vi "Main Tclk.vi"() -> ()   [LabVIEW 2018] (continued)
                      frame 2 {
                        n2570 = local read "Specimen I array"() -> (w7608:sgl[])
                        n2571 = local read "Beam Dump 1 array"() -> (w7591:sgl[])
                        n2572 = local read "Milling I array"() -> (w7579:sgl[])
                        n2573 = call "Auto limits.vi"("Minimum half range"=0.5, "# of interquartile range or stdev"=6.0 ("# of sigma"), "Length"=100, "Input array"=w7608) -> ("Low limit"=w7606:dbl, "High limit"=w7607:dbl)  [unwired: 5 in, 1 out]
                        n2574 = call "Auto limits.vi"("Minimum half range"=0.5, "# of interquartile range or stdev"=6.0 ("# of sigma"), "Length"=100, "Input array"=w7591) -> ("Low limit"=w7593:dbl, "High limit"=w7592:dbl)  [unwired: 5 in, 1 out]
                        n2575 = call "Auto limits.vi"("Minimum half range"=0.5, "# of interquartile range or stdev"=6.0 ("# of sigma"), "Length"=100, "Input array"=w7579) -> ("Low limit"=w7581:dbl, "High limit"=w7580:dbl)  [unwired: 5 in, 1 out]
                        n2576 = To Single Precision Float(number=w7607) -> (single precision float=w7601:sgl)
                        n2577 = To Single Precision Float(number=w7606) -> (single precision float=w7600:sgl)
                        n2578 = To Single Precision Float(number=w7592) -> (single precision float=w7598:sgl)
                        n2579 = To Single Precision Float(number=w7593) -> (single precision float=w7599:sgl)
                        n2580 = To Single Precision Float(number=w7580) -> (single precision float=w7586:sgl)
                        n2581 = To Single Precision Float(number=w7581) -> (single precision float=w7587:sgl)
                        n2582 = local read "Specimen I high limit array"() -> (w7603:sgl[])
                        n2583 = local read "Specimen I low limit array"() -> (w7604:sgl[])
                        n2584 = local read "BD1 high limit array"() -> (w7596:sgl[])
                        n2585 = local read "Milling I high limit array"() -> (w7584:sgl[])
                        n2586 = local read "BD1 low limit array"() -> (w7595:sgl[])
                        n2587 = local read "Milling I low limit array"() -> (w7583:sgl[])
                        n2588 = Build Array (concatenate)(w7603, w7601) -> (w7602:sgl[])
                        n2589 = Build Array (concatenate)(w7604, w7600) -> (w7605:sgl[])
                        n2590 = Build Array (concatenate)(w7596, w7598) -> (w7597:sgl[])
                        n2591 = Build Array (concatenate)(w7595, w7599) -> (w7594:sgl[])
                        n2592 = Build Array (concatenate)(w7584, w7586) -> (w7585:sgl[])
                        n2593 = Build Array (concatenate)(w7583, w7587) -> (w7582:sgl[])
                        n2594 = local write "Specimen I high limit array"(w7602) -> ()
                        n2595 = local write "Specimen I low limit array"(w7605) -> ()
                        n2596 = local write "BD1 high limit array"(w7597) -> ()
                        n2597 = local write "Milling I high limit array"(w7585) -> ()
                        n2598 = local write "BD1 low limit array"(w7594) -> ()
                        n2599 = local write "Milling I low limit array"(w7582) -> ()
                      }
                      frame 3 {
                        n2600 = local read "Specimen I array"() -> (w7644:sgl[])
                        n2601 = local read "Beam Dump 1 array"() -> (w7627:sgl[])
                        n2602 = local read "Beam Dump 2 array"() -> (w7620:sgl[])
                        n2603 = call "Auto limits.vi"("Minimum half range"=0.5, "# of interquartile range or stdev"=6.0 ("# of sigma"), "Length"=100, "Input array"=w7644) -> ("Low limit"=w7642:dbl, "High limit"=w7643:dbl)  [unwired: 5 in, 1 out]
                        n2604 = call "Auto limits.vi"("Minimum half range"=0.5, "# of interquartile range or stdev"=6.0 ("# of sigma"), "Length"=100, "Input array"=w7627) -> ("Low limit"=w7629:dbl, "High limit"=w7628:dbl)  [unwired: 5 in, 1 out]
                        n2605 = call "Auto limits.vi"("Minimum half range"=0.5, "# of interquartile range or stdev"=6.0 ("# of sigma"), "Length"=100, "Input array"=w7620) -> ("Low limit"=w7618:dbl, "High limit"=w7619:dbl)  [unwired: 5 in, 1 out]
                        n2606 = To Single Precision Float(number=w7643) -> (single precision float=w7637:sgl)
                        n2607 = To Single Precision Float(number=w7642) -> (single precision float=w7636:sgl)
                        n2608 = To Single Precision Float(number=w7628) -> (single precision float=w7634:sgl)
                        n2609 = To Single Precision Float(number=w7629) -> (single precision float=w7635:sgl)
                        n2610 = To Single Precision Float(number=w7619) -> (single precision float=w7613:sgl)
                        n2611 = To Single Precision Float(number=w7618) -> (single precision float=w7612:sgl)
                        n2612 = local read "Specimen I high limit array"() -> (w7639:sgl[])
                        n2613 = local read "Specimen I low limit array"() -> (w7640:sgl[])
                        n2614 = local read "BD1 high limit array"() -> (w7632:sgl[])
                        n2615 = local read "BD2 high limit array"() -> (w7615:sgl[])
                        n2616 = local read "BD1 low limit array"() -> (w7631:sgl[])
                        n2617 = local read "BD2 low limit array"() -> (w7616:sgl[])
                        n2618 = Build Array (concatenate)(w7639, w7637) -> (w7638:sgl[])
                        n2619 = Build Array (concatenate)(w7640, w7636) -> (w7641:sgl[])
                        n2620 = Build Array (concatenate)(w7632, w7634) -> (w7633:sgl[])
                        n2621 = Build Array (concatenate)(w7631, w7635) -> (w7630:sgl[])
                        n2622 = Build Array (concatenate)(w7615, w7613) -> (w7614:sgl[])
                        n2623 = Build Array (concatenate)(w7616, w7612) -> (w7617:sgl[])
                        n2624 = local write "Specimen I high limit array"(w7638) -> ()
                        n2625 = local write "Specimen I low limit array"(w7641) -> ()
                        n2626 = local write "BD1 high limit array"(w7633) -> ()
                        n2627 = local write "BD2 high limit array"(w7614) -> ()
                        n2628 = local write "BD1 low limit array"(w7630) -> ()
                        n2629 = local write "BD2 low limit array"(w7617) -> ()
                      }
                      frame 100, Default {
                        n2630 = local read "Specimen I array"() -> (w7692:sgl[])
                        n2631 = local read "Beam Dump 1 array"() -> (w7675:sgl[])
                        n2632 = local read "Beam Dump 2 array"() -> (w7668:sgl[])
                        n2633 = local read "Milling I array"() -> (w7651:sgl[])
                        n2634 = call "Auto limits.vi"("Minimum half range"=0.5, "# of interquartile range or stdev"=6.0 ("# of sigma"), "Length"=100, "Input array"=w7692) -> ("Low limit"=w7690:dbl, "High limit"=w7691:dbl)  [unwired: 5 in, 1 out]
                        n2635 = call "Auto limits.vi"("Minimum half range"=0.5, "# of interquartile range or stdev"=6.0 ("# of sigma"), "Length"=100, "Input array"=w7675) -> ("Low limit"=w7677:dbl, "High limit"=w7676:dbl)  [unwired: 5 in, 1 out]
                        n2636 = call "Auto limits.vi"("Minimum half range"=0.5, "# of interquartile range or stdev"=6.0 ("# of sigma"), "Length"=100, "Input array"=w7668) -> ("Low limit"=w7666:dbl, "High limit"=w7667:dbl)  [unwired: 5 in, 1 out]
                        n2637 = call "Auto limits.vi"("Minimum half range"=0.5, "# of interquartile range or stdev"=6.0 ("# of sigma"), "Length"=100, "Input array"=w7651) -> ("Low limit"=w7653:dbl, "High limit"=w7652:dbl)  [unwired: 5 in, 1 out]
                        n2638 = To Single Precision Float(number=w7691) -> (single precision float=w7685:sgl)
                        n2639 = To Single Precision Float(number=w7690) -> (single precision float=w7684:sgl)
                        n2640 = To Single Precision Float(number=w7676) -> (single precision float=w7682:sgl)
                        n2641 = To Single Precision Float(number=w7677) -> (single precision float=w7683:sgl)
                        n2642 = To Single Precision Float(number=w7667) -> (single precision float=w7661:sgl)
                        n2643 = To Single Precision Float(number=w7666) -> (single precision float=w7660:sgl)
                        n2644 = To Single Precision Float(number=w7652) -> (single precision float=w7658:sgl)
                        n2645 = To Single Precision Float(number=w7653) -> (single precision float=w7659:sgl)
                        n2646 = local read "Specimen I high limit array"() -> (w7687:sgl[])
                        n2647 = local read "Specimen I low limit array"() -> (w7688:sgl[])
                        n2648 = local read "BD1 high limit array"() -> (w7680:sgl[])
                        n2649 = local read "BD2 high limit array"() -> (w7663:sgl[])
                        n2650 = local read "Milling I high limit array"() -> (w7656:sgl[])
                        n2651 = local read "BD1 low limit array"() -> (w7679:sgl[])
                        n2652 = local read "BD2 low limit array"() -> (w7664:sgl[])
                        n2653 = local read "Milling I low limit array"() -> (w7655:sgl[])
                        n2654 = Build Array (concatenate)(w7687, w7685) -> (w7686:sgl[])
                        n2655 = Build Array (concatenate)(w7688, w7684) -> (w7689:sgl[])
                        n2656 = Build Array (concatenate)(w7680, w7682) -> (w7681:sgl[])
                        n2657 = Build Array (concatenate)(w7679, w7683) -> (w7678:sgl[])
                        n2658 = Build Array (concatenate)(w7663, w7661) -> (w7662:sgl[])
                        n2659 = Build Array (concatenate)(w7664, w7660) -> (w7665:sgl[])
                        n2660 = Build Array (concatenate)(w7656, w7658) -> (w7657:sgl[])
                        n2661 = Build Array (concatenate)(w7655, w7659) -> (w7654:sgl[])
                        n2662 = local write "Specimen I high limit array"(w7686) -> ()
                        n2663 = local write "Specimen I low limit array"(w7689) -> ()
                        n2664 = local write "BD1 high limit array"(w7681) -> ()
                        n2665 = local write "BD2 high limit array"(w7662) -> ()
                        n2666 = local write "Milling I high limit array"(w7657) -> ()
                        n2667 = local write "BD1 low limit array"(w7678) -> ()
                        n2668 = local write "BD2 low limit array"(w7665) -> ()
                        n2669 = local write "Milling I low limit array"(w7654) -> ()
                      }
                    }
                  }
                }
                n2670 = local read "Delta X array for stop limit"() -> (w7442:sgl[])
                n2671 = local read "Delta Y array for stop limit"() -> (w7439:sgl[])
                n2672 = local read "X shift (nm/image)"() -> (w7428:sgl)
                n2673 = local read "Y shift (nm/image)"() -> (w7425:sgl)
                n2674 = Absolute Value(x=w7442) -> (abs(x)=w7435:sgl[])
                n2675 = Absolute Value(x=w7439) -> (abs(x)=w7434:sgl[])
                n2676 = local read "Delta X stop limit array"() -> (w7443:sgl[])
                n2677 = local read "Delta Y stop limit array"() -> (w7437:sgl[])
                n2678 = call "Auto limits.vi"("Method"="mean & stdev", "Minimum half range"=10.0 ("# of sigma"), "# of interquartile range or stdev"=6.0 ("# of sigma"), "Length"=10, "Input array"=w7435) -> ("High limit"=w7422:dbl)  [unwired: 4 in, 2 out]
                n2679 = call "Auto limits.vi"("Method"="mean & stdev", "Minimum half range"=10.0 ("# of sigma"), "# of interquartile range or stdev"=6.0 ("# of sigma"), "Length"=100, "Input array"=w7434) -> ("High limit"=w7438:dbl)  [unwired: 4 in, 2 out]
                n2680 = To Single Precision Float(number=w7422) -> (single precision float=w7445:sgl)
                n2681 = To Single Precision Float(number=w7438) -> (single precision float=w7424:sgl)
                n2682 = Absolute Value(x=w7428) -> (abs(x)=w7420:sgl)
                n2683 = Absolute Value(x=w7425) -> (abs(x)=w7421:sgl)
                n2684 = Add(x=w7445, y=w7420) -> (x+y=w7429:sgl)
                n2685 = Add(x=w7424, y=w7421) -> (x+y=w7426:sgl)
                n2686 = Build Array (concatenate)(w7443, w7429) -> (w7444:sgl[])
                n2687 = Build Array (concatenate)(w7437, w7426) -> (w7436:sgl[])
                n2688 = local write "Delta X stop limit array"(w7444) -> ()
                n2689 = local write "Delta Y stop limit array"(w7436) -> ()
              }
              frame #27 {
                n2690 = local read "Pause for reheat"() -> (w7722:bool)
                n2691 = local read "Auto re-engage"() -> (w7721:bool)
                n2692 = case shown="True" w7722 {
                  tunnel: w7721 -> [_ w7723]
                  frame False {
                  }
                  frame True {
                    n2693 = case shown="False" w7723 {
                      frame False {
                        n2694 = stacked-sequence {
                          frame #0 {
                            n2695 = local read "3D FIB-SEM Files"() -> (w7729:path)
                            n2696 = local read "Re-engage Files"() -> (w7732:path)
                            n2697 = Build Path(base path=w7729, name or relative path="LG low res.png " ("command line")) -> (appended path=w7728:path)
                            n2698 = Build Path(base path=w7732, name or relative path="pre.png " ("command line")) -> (appended path=w7727:path)
                            n2699 = Copy(9:TRUE ("run minimized? (F)"), 10:w7727, 11:w7728) -> ()  [unwired: 2 in, 3 out]
                          }
                          frame #1 {
                            n2700 = shared-variable ".\\Zeiss Library.lvlib\\Timestamp"() -> (→"Pre-reheat time":timestamp)  [unwired: 1 in, 1 out]
                            n2701 = local read "Last good FI"() -> (→"Pre-reheat FI":sgl)
                          }
                          frame #2 {
                            n2702 = local read "SEM Scan Parameters"() -> (w7735:T26)
                            n2703 = Unbundle By Name(w7735) -> ("X center (um)"=→"Pre-reheat X center (um)":sgl, "Y center (um)"=→"Pre-reheat Y center (um)":sgl, "Y stig"=w7738:sgl[][])
                            n2704 = local write "Pre-reheat Y stig"(w7738) -> ()
                          }
                        }
                      }
                      frame True {
                      }
                    }
                    n2705 = local write "Mill Manual Pause"(TRUE ("Mill Stop")) -> ()
                    n2706 = property on="Mill Manual Pause" class="Bool (strict)"("DisabledEnum"=T44."Disabled and Grayed Out" ("Disabled")) -> ()  [unwired: 2 in, 2 out]
                  }
                }
              }
              frame #28 {
                n2707 = local read "FIB"() -> (w7747:bool)
                n2708 = local read "Alert Settings"() -> (w7745:T36)
                n2709 = local read "Log time array"() -> (w7740:u32[])
                n2710 = case shown="True" w7747 {
                  frame False {
                  }
                  frame True {
                    n2711 = local read "Temp (F)"() -> (w7798:sgl)
                    n2712 = local read "Faraday Cup (nA)"() -> (w7799:sgl)
                    n2713 = local read "Specimen I (nA)"() -> (w7800:sgl)
                    n2714 = local read "Beam Dump 1 (nA)"() -> (w7801:sgl)
                    n2715 = local read "Beam Dump 2 (nA)"() -> (w7784:sgl)
                    n2716 = local read "Milling I (nA)"() -> (w7783:sgl)
                    n2717 = local read "SEM Specimen I"() -> (w7781:dbl)
                    n2718 = local read "Milling Z voltage (V)"() -> (w7782:sgl)
                    n2719 = local read "File Information"() -> (w7802:T31)
                    n2720 = shared-variable ".\\Zeiss Library.lvlib\\Timestamp"() -> (w7787:timestamp)  [unwired: 1 in, 1 out]
                    n2721 = Unbundle By Name(w7802) -> ("File path"=w7785:path)
                    n2722 = Build Array(w7798, w7799, w7800, w7801, w7784, w7783, w7781, w7782) -> (w7788:dbl[])
                    n2723 = for {
                      tunnel: w7788 -> [w7804] mode=indexing
                      tunnel: [w7803] -> w7789 mode=indexing
                      n2724 = Format Into String(w7804) -> (resulting string=w7803:string)  [unwired: 3 in, 1 out]
                    }
                    n2725 = call "YMD log files.vi"("Input text array"=w7789, "Start new line"=FALSE, "current time"=w7787, "Log file path"=w7785) -> ()  [unwired: 8 in]
                    n2726 = local read "Milling Z voltage array"() -> (w7776:sgl[])
                    n2727 = local read "Last milling snapshot"() -> (w7790:path)
                    n2728 = shared-variable ".\\Zeiss Library.lvlib\\Timestamp"() -> (w7794:timestamp)  [unwired: 1 in, 1 out]
                    n2729 = local read "FIB slice #"() -> (w7792:u32)
                    n2730 = local read "Pause for reheat"() -> (w7795:bool)
                    n2731 = local read "Last good FI"() -> (w7797:sgl)
                    n2732 = local read "Focus Index"() -> (w7796:sgl)
                    n2733 = local read "Hardware Configuration"() -> (w7780:T25)
                    n2734 = Unbundle By Name(w7780) -> ("SEM Max FOV (um)"=w7779:sgl)
                    n2735 = Array Size(array=w7776) -> (size(s)=w7778:i32)
                    n2736 = expression code="x-2"(w7778) -> (w7777:i32)
                    n2737 = Index Array(array=w7776, index=w7777) -> (element=w7775:sgl)
                    n2738 = Bundle("Timestamp"=w7794, "Milling Z voltage (V)"=w7775, "FIB slice #"=w7792, "Pause for reheat"=w7795, "Last good FI"=w7797, "Focus Index"=w7796, "SEM Max FOV (um)"=w7779) -> (w7791:T57)  [unwired: 1 in]
                    n2739 = Flatten To XML(anything=w7791) -> (xml string=w7793:string)
                    n2740 = call-poly <vilib>:"Write to XML File.vi"("XML Input"=w7793, "XML File Path"=w7790) -> ()  [unwired: 7 in, 3 out]
                  }
                }
                n2741 = Unbundle By Name(w7745) -> ("Focus index low limit"=w7744:sgl)
                n2742 = Array Size(array=w7740) -> (size(s)=w7739:i32)
                n2743 = local read "Focus Index"() -> (w7742:sgl)
                n2744 = Greater Than 0?(x=w7739) -> (x > 0?=w7741:bool)
                n2745 = case shown="True" w7741 {
                  tunnel: w7740 -> [_ w7762]
                  frame False {
                    w7748 = T44."Disabled and Grayed Out" ("Disabled")
                    n2746 = property on="Actual cycle time (s)" class="DigNum (strict)"("DisabledEnum"=w7748) -> ()  [unwired: 2 in, 2 out]
                    n2747 = property on="Median cycle time (s)" class="DigNum (strict)"("DisabledEnum"=w7748) -> ()  [unwired: 2 in, 2 out]
                    n2748 = property on="Daily Z removal (um)" class="DigNum (strict)"("DisabledEnum"=w7748) -> ()  [unwired: 2 in, 2 out]
                    n2749 = property on="Median cycle time est offset (s)" class="DigNum (strict)"("DisabledEnum"=w7748) -> ()  [unwired: 2 in, 2 out]
                  }
                  frame True {
                    w7752 = T44."Enabled" ("Disabled")
                    n2750 = local read "Cycle time array"() -> (w7763:u32[])
                    n2751 = shared-variable ".\\Zeiss Library.lvlib\\Timestamp"() -> (w7761:timestamp)  [unwired: 1 in, 1 out]
                    n2752 = Reverse 1D Array(array=w7762) -> (reversed array=w7766:u32[])
                    n2753 = local read "Est. cycle time (s)"() -> (w7750:u32)
                    n2754 = local read "Cycle time est offset array"() -> (w7755:i16[])
                    n2755 = Index Array(array=w7766, index=0) -> (element=w7764:u32)
                    n2756 = To Unsigned Long Integer(number=w7761) -> (unsigned 32bit integer=w7760:u32)
                    n2757 = Subtract(x=w7760, y=w7764) -> (x-y=w7757:u32)
                    "Actual cycle time (s)" <- w7757
                    n2758 = To Word Integer(number=w7750) -> (16bit integer=w7749:i16)
                    n2759 = To Word Integer(number=w7757) -> (16bit integer=w7751:i16)
                    n2760 = Build Array (concatenate)(w7763, w7757) -> (w7759:u32[])
                    n2761 = Subtract(x=w7751, y=w7749) -> (x-y=w7756:i16)
                    n2762 = local write "Cycle time array"(w7759) -> ()
                    n2763 = Build Array (concatenate)(w7755, w7756) -> (w7754:i16[])
                    n2764 = local write "Cycle time est offset array"(w7754) -> ()
                    n2765 = call <vilib>:"Median.vi"("X"=w7754) -> ("median"=→"Median cycle time est offset (s)":dbl)  [unwired: 1 out]
                    n2766 = call <vilib>:"Median.vi"("X"=w7759) -> ("median"=→"Median cycle time (s)":dbl)  [unwired: 1 out]
                    n2767 = property on="Actual cycle time (s)" class="DigNum (strict)"("DisabledEnum"=w7752) -> ()  [unwired: 2 in, 2 out]
                    n2768 = property on="Median cycle time (s)" class="DigNum (strict)"("DisabledEnum"=w7752) -> ()  [unwired: 2 in, 2 out]
                    n2769 = property on="Daily Z removal (um)" class="DigNum (strict)"("DisabledEnum"=w7752) -> ()  [unwired: 2 in, 2 out]
                    n2770 = property on="Median cycle time est offset (s)" class="DigNum (strict)"("DisabledEnum"=w7752) -> ()  [unwired: 2 in, 2 out]
                  }
                }
                n2771 = Greater Or Equal?(x=w7742, y=w7744) -> (x >= y?=w7743:bool)
                n2772 = case shown="True" w7743 {
                  frame False {
                  }
                  frame True {
                    n2773 = local read "3D FIB-SEM Files"() -> (w7770:path)
                    n2774 = Build Path(base path=w7770, name or relative path="Low res.png") -> (appended path=w7769:path)
                    n2775 = Build Path(base path=w7770, name or relative path="LG low res.png") -> (appended path=w7768:path)
                    n2776 = Copy(9:TRUE ("overwrite (F)"), 10:w7768, 11:w7769) -> ()  [unwired: 2 in, 3 out]
                  }
                }
                n2777 = local read "Reheat from last"() -> (w7746:bool)
                n2778 = case shown="True" w7746 {
                  frame False {
                  }
                  frame True {
                    w7773 = TRUE ("Mill Stop")
                    n2779 = local write "Pause for reheat"(w7773) -> ()
                    n2780 = local write "Mill Manual Pause"(w7773) -> ()
                    n2781 = property on="Mill Manual Pause" class="Bool (strict)"("DisabledEnum"=T44."Disabled and Grayed Out" ("Disabled")) -> ()  [unwired: 2 in, 2 out]
                  }
                }
              }
              frame #29 {
                n2782 = local read "Alert Settings"() -> (w7819:T36)
                n2783 = Unbundle By Name(w7819) -> ("Low limit (F)"=w7818:sgl, "High limit (F)"=w7817:sgl)
                n2784 = stacked-sequence {
                  tunnel: w7818 -> [_ w7915 _]
                  tunnel: w7817 -> [_ w7914 _]
                  tunnel: [w7847 _ _] -> w7805
                  frame #0 {
                    n2785 = local read "Log time array"() -> (w7855:u32[])
                    n2786 = shared-variable ".\\Zeiss Library.lvlib\\Timestamp"() -> (w7891:timestamp)  [unwired: 1 in, 1 out]
                    n2787 = local read "Temp array"() -> (w7886:sgl[])
                    n2788 = local read "Temp low limit array"() -> (w7868:sgl[])
                    n2789 = local read "Faraday Cup array"() -> (w7892:sgl[])
                    n2790 = local read "Faraday Cup high limit array"() -> (w7860:sgl[])
                    n2791 = local read "Faraday Cup low limit array"() -> (w7861:sgl[])
                    n2792 = local read "Specimen I high limit array"() -> (w7871:sgl[])
                    n2793 = local read "Specimen I low limit array"() -> (w7870:sgl[])
                    n2794 = local read "SEM Specimen I array"() -> (w7879:sgl[])
                    n2795 = local read "SEM Specimen I low limit array"() -> (w7866:sgl[])
                    n2796 = case shown="2" "Beam dump display" {
                      tunnel: [w7896 w7899 w7902] -> w7874
                      tunnel: [w7895 w7898 w7901] -> w7850
                      tunnel: [w7894 w7897 w7900] -> w7849
                      frame 0, Default {
                        n2797 = local read "Beam Dump 1 array"() -> (w7896:sgl[])
                        n2798 = local read "BD1 high limit array"() -> (w7895:sgl[])
                        n2799 = local read "BD1 low limit array"() -> (w7894:sgl[])
                      }
                      frame 1 {
                        n2800 = local read "Beam Dump 2 array"() -> (w7899:sgl[])
                        n2801 = local read "BD2 high limit array"() -> (w7898:sgl[])
                        n2802 = local read "BD2 low limit array"() -> (w7897:sgl[])
                      }
                      frame 2 {
                        n2803 = local read "Milling I array"() -> (w7902:sgl[])
                        n2804 = local read "Milling I high limit array"() -> (w7901:sgl[])
                        n2805 = local read "Milling I low limit array"() -> (w7900:sgl[])
                      }
                    }
                    n2806 = local read "Focus index array"() -> (w7887:sgl[])
                    n2807 = local read "FI low limit array"() -> (w7872:sgl[])
                    n2808 = local read "Temp high limit array"() -> (w7869:sgl[])
                    n2809 = local read "Specimen I array"() -> (w7893:sgl[])
                    n2810 = local read "SEM Specimen I high limit array"() -> (w7867:sgl[])
                    n2811 = To Unsigned Long Integer(number=w7891) -> (unsigned 32bit integer=w7854:u32)
                    n2812 = Build Array (concatenate)(w7855, w7854) -> (w7847:u32[])
                    n2813 = Bundle(w7847, "Faraday Cup high limit array"=w7860) -> (w7858:T58)  [unwired: 1 in]
                    n2814 = Bundle(w7847, "Faraday Cup low limit array"=w7861) -> (w7859:T59)  [unwired: 1 in]
                    n2815 = Bundle(w7847, "SEM Specimen I array"=w7879) -> (w7864:cluster{u32[], "SEM Specimen I array":sgl[]})  [unwired: 1 in]
                    n2816 = Bundle(w7847, "SEM Specimen I high limit array"=w7867) -> (w7865:T60)  [unwired: 1 in]
                    n2817 = local write "Log time array"(w7847) -> ()
                    n2818 = Bundle(w7847, "Temp array"=w7886) -> (w7884:cluster{u32[], "Temp array":sgl[]})  [unwired: 1 in]
                    n2819 = Bundle(w7847, "Temp high limit array"=w7869) -> (w7885:cluster{u32[], "Temp high limit array":sgl[]})  [unwired: 1 in]
                    n2820 = Bundle(w7847, "Temp low limit array"=w7868) -> (w7883:cluster{u32[], "Temp low limit array":sgl[]})  [unwired: 1 in]
                    n2821 = Bundle(w7847, "Faraday Cup array"=w7892) -> (w7857:cluster{u32[], "Faraday Cup array":sgl[]})  [unwired: 1 in]
                    n2822 = Bundle(w7847, "Specimen I high limit array"=w7871) -> (w7877:T61)  [unwired: 1 in]
                    n2823 = Bundle(w7847, "Specimen I low limit array"=w7870) -> (w7878:T62)  [unwired: 1 in]
                    n2824 = Bundle(w7847, "SEM Specimen I low limit array"=w7866) -> (w7863:T63)  [unwired: 1 in]
                    n2825 = Bundle(w7847, "Milling I array"=w7874) -> (w7851:cluster{u32[], "Milling I array":sgl[]})  [unwired: 1 in]
                    n2826 = Bundle(w7847, "Milling I high limit array"=w7850) -> (w7853:T64)  [unwired: 1 in]
                    n2827 = Bundle(w7847, "Milling I low limit array"=w7849) -> (w7852:T65)  [unwired: 1 in]
                    n2828 = Bundle(w7847, "Focus index array"=w7887) -> (w7890:cluster{u32[], "Focus index array":sgl[]})  [unwired: 1 in]
                    n2829 = Bundle(w7847, "FI low limit array"=w7872) -> (w7889:cluster{u32[], "FI low limit array":sgl[]})  [unwired: 1 in]
                    n2830 = Bundle(w7847, "Specimen I array"=w7893) -> (w7876:cluster{u32[], "Specimen I array":sgl[]})  [unwired: 1 in]
                    n2831 = Build Array(w7857, w7858, w7859) -> (→"Faraday Cup log":T66)
                    n2832 = Build Array(w7884, w7885, w7883) -> (→"Temp log":cluster{u32[], "Temp low limit array":sgl[]}[])
                    n2833 = Build Array(w7876, w7877, w7878) -> (w7875:T67)
                    n2834 = Build Array(w7864, w7865, w7863) -> (w7862:T68)
                    n2835 = Build Array(w7851, w7853, w7852) -> (→"Beam Dump log":T69)
                    n2836 = Build Array(w7890, w7889) -> (→"Focus index log":cluster{u32[], "FI low limit array":sgl[]}[])
                    n2837 = Select(t=w7875, s="Specimen current toggle", f=w7862) -> (s? t:f=→"Specimen I log":T68)
                  }
                  frame #1 {
                    n2838 = local read "Delta Z mode"() -> (w7912:u8)
                    n2839 = expression code="x-0.2"(w7915) -> (w7916:sgl)
                    n2840 = expression code="x+0.2"(w7914) -> (w7917:sgl)
                    n2841 = property on="Temp log" class="XYGraph (strict)"("YScale.Minimum"=w7916) -> ()  [unwired: 2 in, 2 out]
                    n2842 = property on="Temp log" class="XYGraph (strict)"("YScale.Maximum"=w7917) -> ()  [unwired: 2 in, 2 out]
                    n2843 = case shown="2" w7912 {
                      tunnel: [w7920 w7921 w7922] -> w7903
                      frame 0, Default {
                        n2844 = local read "Delta image array"() -> (w7920:sgl[])
                      }
                      frame 1 {
                        n2845 = local read "Delta Z array"() -> (w7921:sgl[])
                      }
                      frame 2 {
                        n2846 = local read "Milling Z voltage array"() -> (w7922:sgl[])
                      }
                    }
                    n2847 = Array Subset(array=w7903, index=1) -> (w7906:sgl[])  [unwired: 1 in]
                    n2848 = property on="Focus index log" class="XYGraph (strict)"() -> ("XScale.Range"=w7913:T70)  [unwired: 2 in, 2 out]
                    n2849 = Array Size(array=w7906) -> (size(s)=w7904:i32)
                    n2850 = call "Auto limits.vi"("Minimum half range"=0.2, "# of interquartile range or stdev"=1.5 ("# of sigma"), "Input array"=w7906) -> ("Low limit"=w7911:dbl, "High limit"=w7910:dbl)  [unwired: 6 in, 1 out]
                    n2851 = Not Equal To 0?(x=w7904) -> (x != 0?=w7905:bool)
                    n2852 = case shown="True" w7905 {
                      tunnel: w7910 -> [_ w7919]
                      tunnel: w7911 -> [_ w7918]
                      frame False {
                      }
                      frame True {
                        n2853 = property on="Delta Z log" class="XYGraph (strict)"("YScale.Maximum"=w7919) -> ()  [unwired: 2 in, 2 out]
                        n2854 = property on="Delta Z log" class="XYGraph (strict)"("YScale.Minimum"=w7918) -> ()  [unwired: 2 in, 2 out]
                      }
                    }
                    n2855 = property on="Delta X log" class="XYGraph (strict)"("XScale.Range"=w7913) -> ()  [unwired: 2 in, 2 out]
                    n2856 = property on="Delta Y log" class="XYGraph (strict)"("XScale.Range"=w7913) -> ()  [unwired: 2 in, 2 out]
                    n2857 = property on="Delta Z log" class="XYGraph (strict)"("XScale.Range"=w7913) -> ()  [unwired: 2 in, 2 out]
                  }
                  frame #2 {
                    w7926 = T71 {"Left"=658, "Top"=662, "Right"=1206, "Bottom"=800} ("Plot Area Bounds 3")
                    w7925 = T71 {"Left"=658, "Top"=519, "Right"=1206, "Bottom"=657} ("Plot Area Bounds 2")
                    w7924 = T71 {"Left"=658, "Top"=375, "Right"=1206, "Bottom"=513} ("Plot Area Bounds")
                    w7923 = T71 {"Left"=658, "Top"=231, "Right"=1206, "Bottom"=369} ("Plot Area Bounds")
                    n2858 = property on="Temp log" class="XYGraph (strict)"("Plot Bounds"=w7923) -> ()  [unwired: 2 in, 2 out]
                    n2859 = property on="Focus index log" class="XYGraph (strict)"("Plot Bounds"=w7923) -> ()  [unwired: 2 in, 2 out]
                    n2860 = property on="Faraday Cup log" class="XYGraph (strict)"("Plot Bounds"=w7924) -> ()  [unwired: 2 in, 2 out]
                    n2861 = property on="Delta X log" class="XYGraph (strict)"("Plot Bounds"=w7924) -> ()  [unwired: 2 in, 2 out]
                    n2862 = property on="Specimen I log" class="XYGraph (strict)"("Plot Bounds"=w7925) -> ()  [unwired: 2 in, 2 out]
                    n2863 = property on="Delta Y log" class="XYGraph (strict)"("Plot Bounds"=w7925) -> ()  [unwired: 2 in, 2 out]
                    n2864 = property on="Beam Dump log" class="XYGraph (strict)"("Plot Bounds"=w7926) -> ()  [unwired: 2 in, 2 out]
                    n2865 = property on="Delta Z log" class="XYGraph (strict)"("Plot Bounds"=w7926) -> ()  [unwired: 2 in, 2 out]
                  }
                }
                n2866 = case shown="0, Default" "Delta Z mode" {
                  tunnel: [w7844 w7845 w7846] -> w7814
                  frame 0, Default {
                    n2867 = local read "Delta image array"() -> (w7844:sgl[])
                  }
                  frame 1 {
                    n2868 = local read "Delta Z array"() -> (w7845:sgl[])
                  }
                  frame 2 {
                    n2869 = local read "Milling Z voltage array"() -> (w7846:sgl[])
                  }
                }
                n2870 = local read "Delta X array"() -> (w7807:sgl[])
                n2871 = local read "Delta X sum array"() -> (w7806:sgl[])
                n2872 = local read "Delta Y array"() -> (w7808:sgl[])
                n2873 = local read "Delta Y sum array"() -> (w7809:sgl[])
                n2874 = case shown="True" "Delta X toggle" {
                  tunnel: [w7832 w7840] -> w7813
                  tunnel: w7807 -> [_ w7839]
                  tunnel: w7805 -> [w7834 w7838]
                  tunnel: w7806 -> [w7833 _]
                  frame False {
                    n2875 = Bundle(w7834, "Delta X sum array"=w7833) -> (w7835:cluster{u32[], "Delta X sum array":sgl[]})  [unwired: 1 in]
                    n2876 = Build Array(w7835) -> (w7832:cluster{u32[], "Delta X sum array":sgl[]}[])
                  }
                  frame True {
                    n2877 = local read "Delta X stop limit array"() -> (w7836:sgl[])
                    n2878 = Negate(x=w7836) -> (-x=w7837:sgl[])
                    n2879 = Bundle(w7838, "Delta X array"=w7839) -> (w7843:cluster{u32[], "Delta X array":sgl[]})  [unwired: 1 in]
                    n2880 = Bundle(w7838, "Delta X stop limit array"=w7836) -> (w7841:cluster{u32[], "Delta X stop limit array":sgl[]})  [unwired: 1 in]
                    n2881 = Bundle(w7838, w7837) -> (w7842:cluster{u32[], sgl[]})  [unwired: 1 in]
                    n2882 = Build Array(w7843, w7841, w7842) -> (w7840:T72)
                  }
                }
                "Delta X log" <- w7813
                n2883 = case shown="True" "Delta Y toggle" {
                  tunnel: [w7820 w7828] -> w7810
                  tunnel: w7808 -> [_ w7827]
                  tunnel: w7805 -> [w7822 w7826]
                  tunnel: w7809 -> [w7821 _]
                  frame False {
                    n2884 = Bundle(w7822, "Delta Y sum array"=w7821) -> (w7823:cluster{u32[], "Delta Y sum array":sgl[]})  [unwired: 1 in]
                    n2885 = Build Array(w7823) -> (w7820:cluster{u32[], "Delta Y sum array":sgl[]}[])
                  }
                  frame True {
                    n2886 = local read "Delta Y stop limit array"() -> (w7824:sgl[])
                    n2887 = Negate(x=w7824) -> (-x=w7825:sgl[])
                    n2888 = Bundle(w7826, "Delta Y array"=w7827) -> (w7831:cluster{u32[], "Delta Y array":sgl[]})  [unwired: 1 in]
                    n2889 = Bundle(w7826, "Delta Y stop limit array"=w7824) -> (w7829:cluster{u32[], "Delta Y stop limit array":sgl[]})  [unwired: 1 in]
                    n2890 = Bundle(w7826, w7825) -> (w7830:cluster{u32[], sgl[]})  [unwired: 1 in]
                    n2891 = Build Array(w7831, w7829, w7830) -> (w7828:T73)
                  }
                }
                "Delta Y log" <- w7810
                n2892 = Bundle(w7805, "Milling Z voltage array"=w7814) -> (→"Delta Z log":cluster{u32[], "Milling Z voltage array":sgl[]})  [unwired: 1 in]
              }
              frame #30 {
                n2893 = local read "3D FIB-SEM Files"() -> (w7927:path)
                n2894 = local read "SEM Scan Parameters"() -> (w7934:T26)
                n2895 = Unbundle By Name(w7934) -> ("Y tiles"=w7940:u8, "X tiles"=w7941:u8)
                n2896 = Decrement(x=w7940) -> (x-1=w7938:u8)
                n2897 = Decrement(x=w7941) -> (x-1=w7939:u8)
                n2898 = Format Into String(w7938) -> (resulting string=w7935:string)  [unwired: 3 in, 1 out]
                n2899 = Format Into String(w7939) -> (resulting string=w7937:string)  [unwired: 3 in, 1 out]
                n2900 = Concatenate Strings("Primary_grid_" ("name or relative path"), w7935, "-" ("name or relative path"), w7937, ".png" ("name or relative path")) -> (w7929:string)
                n2901 = Build Path(base path=w7927, name or relative path=w7929) -> (appended path=w7930:path)
                n2902 = File/Directory Info(path=w7930) -> (error out=w7931:errorcluster)  [unwired: 1 in, 6 out]
                n2903 = Unbundle By Name(w7931) -> ("status"=w7928:bool)
                n2904 = case shown="False" w7928 {
                  tunnel: w7927 -> [w7942 _]
                  frame False {
                    n2905 = local read "SEM Scan Parameters"() -> (w7945:T26)
                    n2906 = Unbundle By Name(w7945) -> ("Y tiles"=w7944:u8, "X tiles"=w7943:u8)
                    n2907 = for {
                      N: w7944 -> [_]
                      tunnel: w7942 -> [w7947]
                      tunnel: w7943 -> [w7946]
                      i -> [w7948]
                      n2908 = for {
                        N: w7946 -> [_]
                        tunnel: w7948 -> [w7957]
                        tunnel: w7947 -> [w7952]
                        i -> [w7958]
                        n2909 = Format Into String(w7957) -> (resulting string=w7961:string)  [unwired: 3 in, 1 out]
                        n2910 = Format Into String(w7958) -> (resulting string=w7963:string)  [unwired: 3 in, 1 out]
                        n2911 = Concatenate Strings(w7961, "-" ("name or relative path"), w7963, ".png" ("name or relative path")) -> (w7955:string)
                        n2912 = Concatenate Strings("Primary_grid_" ("command line"), w7955) -> (w7954:string)
                        n2913 = Concatenate Strings("post_" ("name or relative path"), w7955) -> (w7953:string)
                        n2914 = Build Path(base path=w7952, name or relative path=w7954) -> (appended path=w7950:path)
                        n2915 = Build Path(base path=w7952, name or relative path=w7953) -> (appended path=w7951:path)
                        n2916 = Move(source path=w7950, 9:TRUE ("run minimized? (F)"), 10:w7951) -> ()  [unwired: 2 in, 3 out]
                      }
                    }
                  }
                  frame True {
                  }
                }
              }
              frame #31 {
                n2917 = local read "FI grid array tiled"() -> (w7974:sgl[][][][][])
                n2918 = local read "WD array tiled"() -> (w7967:sgl[][][])
                n2919 = local read "FI array tiled"() -> (w7968:sgl[][][])
                n2920 = local read "AF Count"() -> (w7969:u8)
                n2921 = local read "AF Steps"() -> (w7971:u8)
                n2922 = local read "Skip Steps tiled"() -> (w7970:u8[][])
                n2923 = local read "Auto Focus"() -> (w7972:bool)
                n2924 = Empty Array?(array=w7967) -> (empty?=w7966:bool)
                n2925 = Not(x=w7972) -> (.not. x?=w7973:bool)
                n2926 = local read "Focus Index Options"() -> (w7965:T28)
                n2927 = Unbundle By Name(w7965) -> ("Keep aspect ratio"=w7964:bool)
                n2928 = case shown="False" w7966 {
                  tunnel: w7967 -> [w7992 _]
                  tunnel: w7968 -> [w7991 _]
                  tunnel: w7969 -> [w7990 _]
                  tunnel: w7970 -> [w7989 _]
                  tunnel: w7971 -> [w7988 _]
                  tunnel: w7973 -> [w7982 _]
                  tunnel: w7974 -> [w7980 _]
                  tunnel: w7964 -> [w7975 _]
                  frame False {
                    n2929 = for {
                      tunnel: w7992 -> [w8016] mode=indexing
                      tunnel: w7991 -> [w8015] mode=indexing
                      tunnel: w7990 -> [w8014]
                      tunnel: w7989 -> [w8013] mode=indexing
                      tunnel: w7988 -> [w8012]
                      tunnel: [w8011] -> w7987 mode=indexing
                      tunnel: [w8009] -> w7986 mode=indexing
                      tunnel: [w8008] -> w7985 mode=indexing
                      tunnel: [w8007] -> w7984 mode=indexing
                      tunnel: [w8006] -> w7983 mode=indexing
                      tunnel: w7982 -> [w8005]
                      tunnel: [w8004] -> w7981 mode=indexing
                      tunnel: w7980 -> [w8003] mode=indexing
                      tunnel: [w8002] -> w7979 mode=indexing
                      tunnel: [w8001] -> w7977 mode=indexing
                      tunnel: [w8000] -> w7976 mode=indexing
                      tunnel: w7975 -> [w7999]
                      i -> [w8010]
                      n2930 = for {
                        tunnel: w8016 -> [w8035] mode=indexing
                        tunnel: w8015 -> [w8034] mode=indexing
                        tunnel: w8014 -> [w8033]
                        tunnel: w8013 -> [w8032] mode=indexing
                        tunnel: w8012 -> [w8031]
                        tunnel: [w8030] -> w8011 mode=indexing
                        tunnel: w8010 -> [w8029]
                        tunnel: [w8027] -> w8009 mode=indexing
                        tunnel: [w8026] -> w8008 mode=indexing
                        tunnel: [w8025] -> w8007 mode=indexing
                        tunnel: [w8024] -> w8006 mode=indexing
                        tunnel: w8005 -> [w8023]
                        tunnel: [w8022] -> w8004 mode=indexing
                        tunnel: w8003 -> [w8021] mode=indexing
                        tunnel: [w8020] -> w8002 mode=indexing
                        tunnel: [w8019] -> w8001 mode=indexing
                        tunnel: [w8018] -> w8000 mode=indexing
                        tunnel: w7999 -> [w8017]
                        i -> [w8028]
                        n2931 = stacked-sequence {
                          seq-local: [w8043 _ _] -> [_ w8085 _]
                          seq-local: [w8037 _ _] -> [_ w8077 _]
                          seq-local: [w8036 _ _] -> [_ w8074 _]
                          tunnel: w8035 -> [w8048 w8075 w8171]
                          tunnel: w8034 -> [w8047 w8089 w8170]
                          tunnel: w8033 -> [w8045 w8071 _]
                          tunnel: w8032 -> [w8042 _ _]
                          tunnel: w8031 -> [w8044 w8069 _]
                          tunnel: [_ w8086 _] -> w8030
                          tunnel: w8029 -> [_ w8084 _]
                          tunnel: w8028 -> [_ w8083 _]
                          tunnel: [w8036 _ _] -> w8027
                          tunnel: [_ w8082 _] -> w8026
                          tunnel: [_ w8081 _] -> w8025
                          tunnel: [_ w8080 _] -> w8024
                          tunnel: w8023 -> [_ w8079 _]
                          tunnel: [_ w8078 _] -> w8022
                          tunnel: w8021 -> [w8038 _ _]
                          tunnel: [_ w8076 _] -> w8020
                          tunnel: [_ w8073 _] -> w8019
                          tunnel: [_ _ w8169] -> w8018
                          tunnel: w8017 -> [_ w8068 _]
                          frame #0 {
                            n2932 = Subtract(x=w8044, y=w8042) -> (x-y=w8046:u8)
                            n2933 = Less?(x=w8045, y=w8046) -> (x < y?=w8049:bool)
                            n2934 = call-poly "Transpose 3D Array.vi"("Transpose"=T51."Pages and Rows", "Input Array"=w8038) -> ("Output Array"=w8039:dbl[][][])  [unwired: 8 in, 1 out]
                            n2935 = case shown="True" w8049 {
                              tunnel: w8048 -> [w8051 w8056]
                              tunnel: w8045 -> [_ w8055]
                              tunnel: w8047 -> [_ w8057]
                              tunnel: [w8051 w8054] -> w8043
                              tunnel: w8042 -> [w8050 w8053]
                              tunnel: [w8050 w8052] -> w8036
                              frame False {
                              }
                              frame True {
                                n2936 = Index Array(array=w8056, index=w8055) -> (element=w8059:sgl)
                                n2937 = call "1D Parabolic Max.vi"("Y"=w8057, "Xt"=w8059, "X"=w8056) -> ("Y(Xt) < Ymin"=w8058:bool)  [unwired: 1 in, 7 out]
                                n2938 = case shown="True" w8058 {
                                tunnel: w8055 -> [_ w8065]
                                tunnel: w8056 -> [w8061 w8066]
                                tunnel: w8053 -> [w8060 w8063]
                                tunnel: [w8061 w8064] -> w8054
                                tunnel: [w8060 w8062] -> w8052
                                frame False {
                                }
                                frame True {
                                n2939 = Delete From Array(array=w8066, length=1, index=w8065) -> (array with subset deleted=w8064:sgl[])  [unwired: 1 out]
                                n2940 = Increment(x=w8063) -> (x+1=w8062:u8)
                                }
                                }
                              }
                            }
                            n2941 = call-poly "Transpose 3D Array.vi"("Transpose"=T51."Rows and Columns", "Input Array"=w8039) -> ("Output Array"=w8037:dbl[][][])  [unwired: 8 in, 1 out]
                          }
                          frame #1 {
                            n2942 = Subtract(x=w8069, y=w8074) -> (x-y=w8072:u8)
                            n2943 = call "1D Parabolic Max.vi"("Y"=w8089, "X"=w8075) -> ("Found max"=w8080:bool, "Ymax"=w8087:dbl, "Xmax"=w8090:dbl, "Finer Best Polynomial Fit"=w8092:dbl[], "Finer X"=w8088:dbl[])  [unwired: 2 in, 3 out]
                            n2944 = Greater Or Equal?(x=w8071, y=w8072) -> (x >= y?=w8091:bool)
                            n2945 = Subtract(x=w8069, y=w8071) -> (x-y=w8070:u8)
                            n2946 = Compound Arithmetic op=OR(w8080, w8091, w8079) -> (w8078:bool)
                            n2947 = case shown="True" w8078 {
                              tunnel: w8090 -> [_ w8143]
                              tunnel: w8089 -> [w8094 w8155]
                              tunnel: w8085 -> [w8102 _]
                              tunnel: w8092 -> [_ w8154]
                              tunnel: w8088 -> [_ w8153]
                              tunnel: w8087 -> [_ w8144]
                              tunnel: w8070 -> [_ w8152]
                              tunnel: w8071 -> [_ w8150]
                              tunnel: [w8102 w8149] -> w8086
                              tunnel: w8084 -> [w8099 w8109]
                              tunnel: w8083 -> [w8100 w8108]
                              tunnel: [w8093 w8144] -> w8082
                              tunnel: [w8097 w8143] -> w8081
                              tunnel: w8077 -> [_ w8135]
                              tunnel: [_ w8134] -> w8076
                              tunnel: w8075 -> [w8098 w8126]
                              tunnel: [w8101 w8125] -> w8073
                              tunnel: w8068 -> [_ w8113]
                              frame False {
                                n2948 = Build Cluster Array(w8098, w8094) -> (w8103:cluster{"Center":sgl, "A Img Focus Index":sgl}[])
                                n2949 = Sort 1D Array(array=w8103) -> (sorted array=w8104:cluster{"Center":sgl, "A Img Focus Index":sgl}[])
                                n2950 = Bundle(w8104) -> (w8105:T74)  [unwired: 1 in]
                                n2951 = Build Array(w8105) -> (w8101:T75)
                                n2952 = local write "AF Y tile"(w8099) -> ()
